vi "addCmdProj.vi"(0 "num_cmd":string, 1 "description":string, 2 "quantite":string, 3 "status_liv":string, 4 "nom_pre_client":string, 5 "tele_client":string, 6 "adresse_client":string, 7 "date_commande":string, 8 "date_livraison":string, 9 "nom_produit":string, 10 "id produit":string, 11 "?":bool) -> ()   [LabVIEW 2024]
uses:
  <vilib>/drjdpowell/SQLite Library/SQL Connection/Open (string).vi
  <vilib>/drjdpowell/SQLite Library/SQL Connection/Execute SQL.vi
  <vilib>/drjdpowell/SQLite Library/SQL Connection/Connection.lvclass
  <vilib>/drjdpowell/SQLite Library/SQLite.lvlib
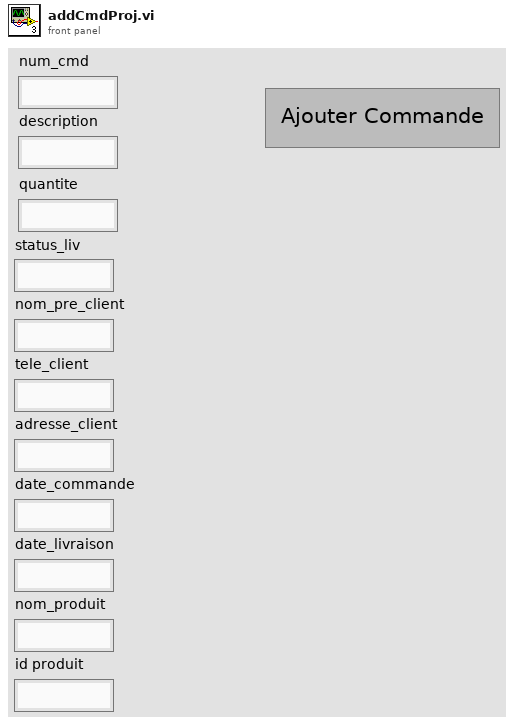
[diagram p1: front panel]
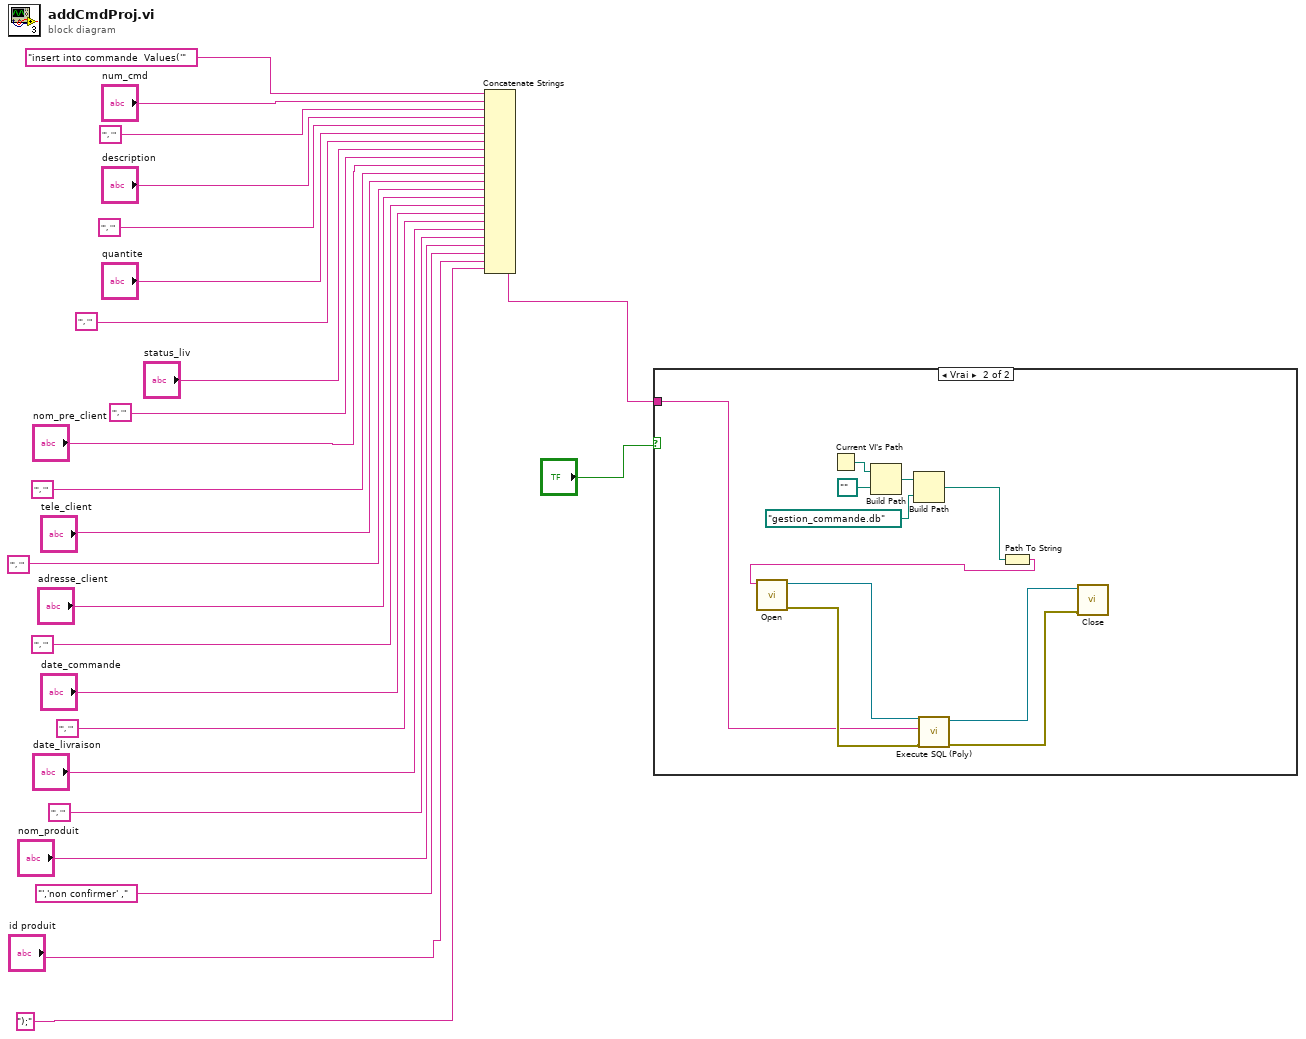
[diagram p0: block diagram]
diagram:
  n1 = Concatenate Strings("insert into commande  Values('", "num_cmd", "', '", "description", "', '", "quantite", "', '", "status_liv", "', '", "nom_pre_client", "', '", "tele_client", "', '", "adresse_client", "', '", "date_commande", "', '", "date_livraison", "', '", "nom_produit", "','non confirmer' ,", "id produit", ");") -> (w1:string)
  n2 = case shown="Vrai" "?" {
    tunnel: w1 -> [_ w32]
    frame False {
    }
    frame True {
      n3 = Current VI's Path() -> (path=w31:path)
      n4 = Build Path(base path=w31, name or relative path=path "..") -> (appended path=w28:path)
      n5 = Build Path(base path=w28, name or relative path=path "gestion_commande.db" ("Filename")) -> (appended path=w27:path)
      n6 = Path To String(path=w27) -> (string=w26:string)
      n7 = call-poly <vilib>:"Open.vi"("db file"=w26) -> ("error out"=w36:errorcluster, "SQLite Connection"=w33:refnum<class "Connection.lvclass">)  [unwired: 9 in]
      n8 = call-poly <vilib>:"Execute SQL (Poly).vi"("error in (no error)"=w36, "SQL"=w32, "SQLite Connection in"=w33) -> ("error out"=w35:errorcluster, "SQLite Connection"=w34:refnum<class "Connection.lvclass">)  [unwired: 5 in, 2 out]
      n9 = call-dynamic "Close.vi"("error in (no error)"=w35, "SQLite Connection in"=w34) -> ()  [unwired: 9 in, 1 out]
    }
  }
